vi "Standardize Delimiters.vi"(8 "error in (no error)":errorcluster, 11 "Command In":string) -> (0 "error out":errorcluster, 3 "Command Out":string)   [LabVIEW 2019, in "PathCommands.lvclass"]
uses:
  PathCommands.lvclass
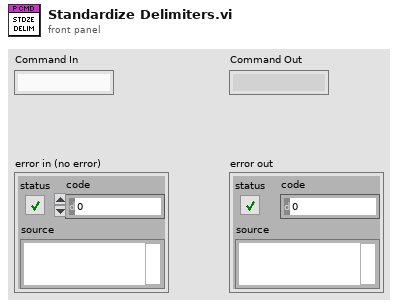
[diagram p1: front panel]
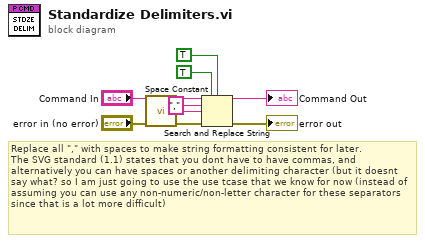
[diagram p0: block diagram]
diagram:
  # "Replace all \",\" with spaces to make string formatting consistent for later.\nThe SVG standard (1.1) states that you dont have to have commas, and alternatively you can have spaces or another delimiting character (but it doesnt say what? so I am just going to use the use tcase that we know for now (instead of assuming you can use any non-numeric/non-letter character for these separators since that is a lot more difficult)"
  n1 = call <vilib>:"Space Constant.vi"() -> ("String"=w5:string)
  n2 = Search and Replace String(replace all?=TRUE ("replace all? (F)"), case sensitive?=TRUE ("ignore case? (F)"), input string="Command In", search string=",", replace string=w5, error in="error in (no error)") -> (result string=→"Command Out":string, error out=→"error out":errorcluster)  [unwired: 2 in, 2 out]
